vi "TcpServer.vi"(10 "Port in (0)":u16, 11 "IpAddress (127.0.0.1)":string="127.0.0.1") -> (0 "error out":errorcluster, 2 "Log":string, 3 "Port out":u16)   [LabVIEW 2022 SP3]
uses:
  TcpSocket/TcpServer/TcpServer.lvclass
  TcpSocket/Connection/Connection.lvclass
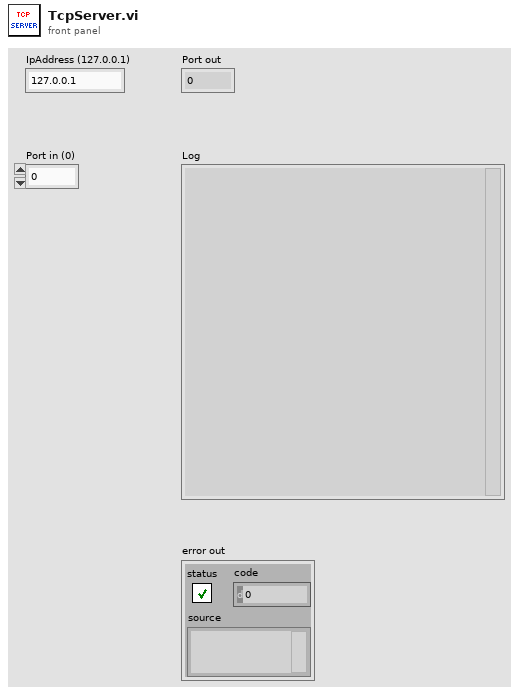
[diagram p1: front panel]
types:
  T1 = enum16{"Standard", "Buffered", "CRLF", "Immediate"}
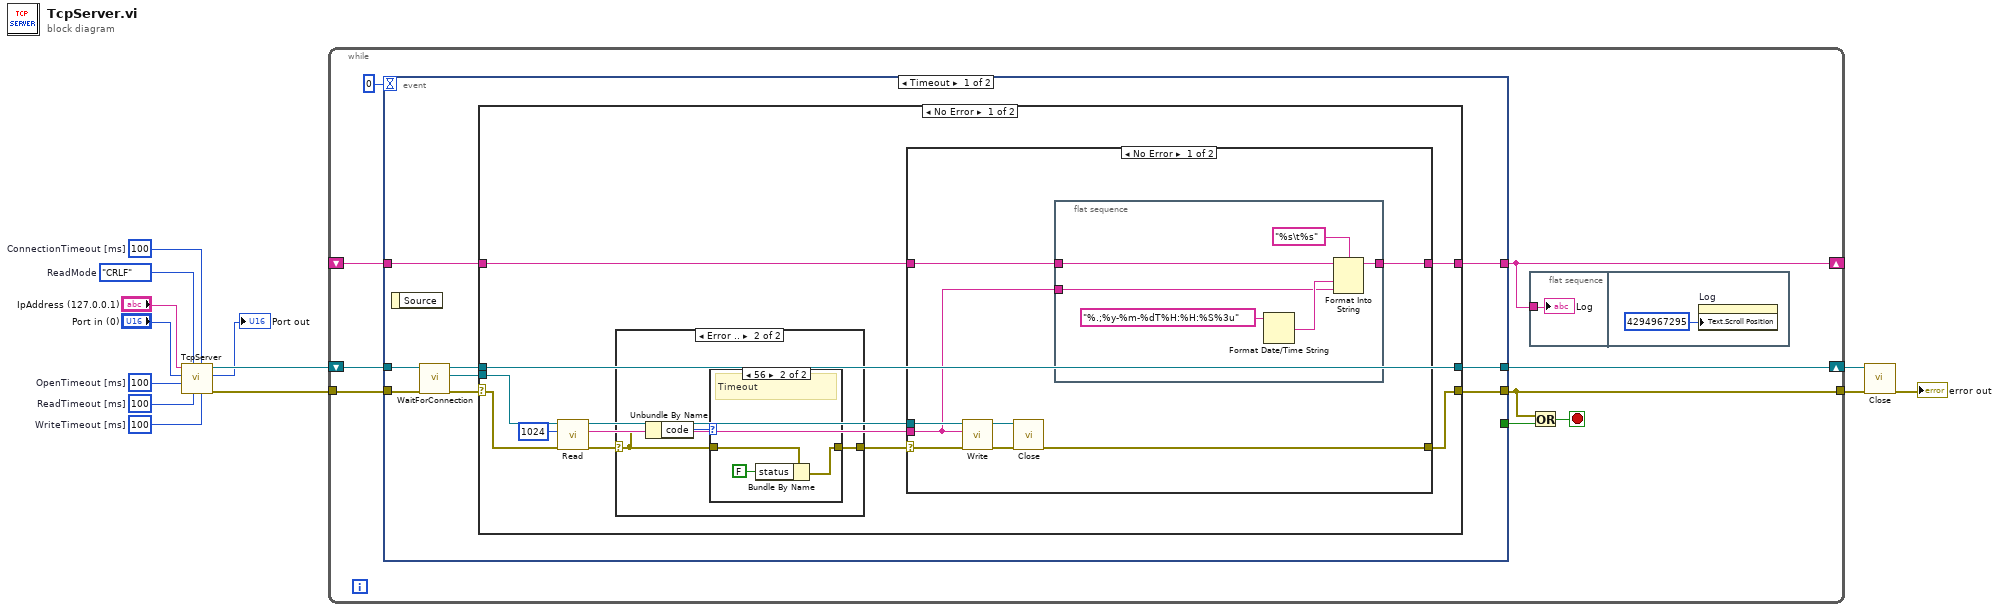
[diagram p0: block diagram]
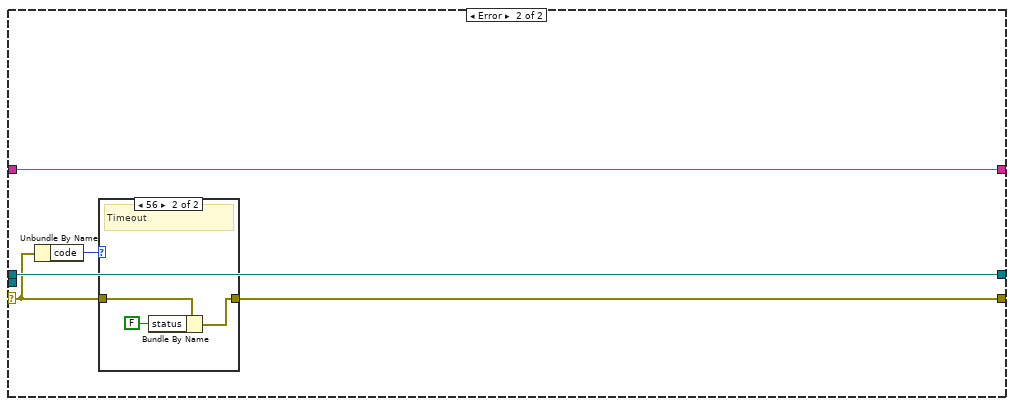
[diagram p5: hidden frame]
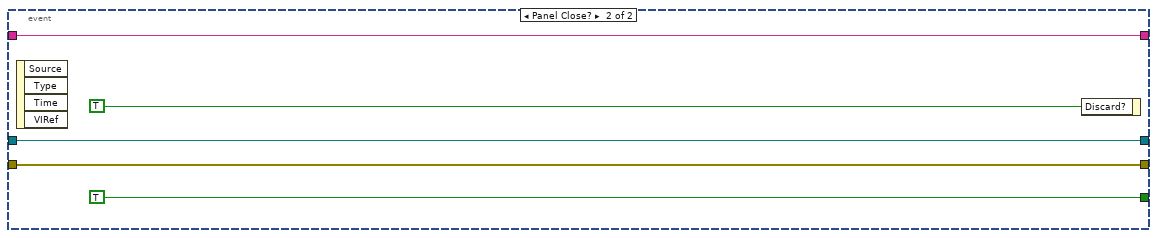
[diagram p7: hidden frame]
diagram:
  w1 = 100  # WriteTimeout [ms]
  w3 = 100  # ReadTimeout [ms]
  w6 = 100  # OpenTimeout [ms]
  w2 = 100  # ConnectionTimeout [ms]
  w7 = T1."CRLF"  # ReadMode
  n1 = call "TcpServer.vi"("WriteTimeout [ms] (5000)"=w1, "ConnectionTimeout [ms] (5000)"=w2, "ReadTimeout [ms] (5000)"=w3, "ReadMode (Standard)"=w7, "OpenTimeout [ms] (5000)"=w6, "Port in (0)"="Port in (0)", "IpAddress (127.0.0.1)"="IpAddress (127.0.0.1)") -> ("error out"=w11:errorcluster, "Port out"=→"Port out":u16, "TcpServer"=w5:refnum<class "TcpServer.lvclass">)  [unwired: 2 in]
  n2 = while {
    tunnel: w11 -> [w22]
    shift-right: [w20] -> w8
    shift-left: w5 -> [w21]
    tunnel: [w17] -> w10
    shift-right: [w14] -> _
    shift-left: _ -> [w15]
    stop <- w18 stop-if-true
    n3 = event shown="[0] Timeout" {
      selector: _ -> [_ _]
      dyn-events: _ -> [_ _]
      timeout: 0 -> [_ _]
      tunnel: w22 -> [w33 w81]
      tunnel: w21 -> [w32 w82]
      tunnel: [w30 w82] -> w20
      tunnel: [w28 w81] -> w17
      tunnel: [_ TRUE] -> w19
      tunnel: w15 -> [w27 w78]
      tunnel: [w26 w78] -> w14
      event Timeout {
        n4 = event-data() -> ()  [unwired: 1 in, 1 out]
        n5 = call-dynamic "WaitForConnection.vi"("error in (no error)"=w33, "TcpServer in"=w32) -> ("error out"=w25:errorcluster, "Connection"=w31:refnum<class "Connection.lvclass">, "TcpServer out"=w29:refnum<class "TcpServer.lvclass">)  [unwired: 7 in]
        n6 = case shown="No Error" w25 {
          selector: w25 -> [w40 w70]
          tunnel: w31 -> [w42 _]
          tunnel: [w44 w73] -> w30
          tunnel: w29 -> [w44 w73]
          tunnel: [w43 w69] -> w28
          tunnel: w27 -> [w36 w72]
          tunnel: [w37 w72] -> w26
          frame No Error {
            n7 = call-dynamic "Read.vi"("error in (no error)"=w40, "BytesToRead"=1024, "Connection in"=w42) -> ("error out"=w35:errorcluster, "Data"=w39:string, "Connection out"=w41:refnum<class "Connection.lvclass">)  [unwired: 6 in]
            n8 = case shown="Error .." w35 {
              selector: w35 -> [w61 w63]
              tunnel: [w61 w62] -> w34
              frame No Error {
              }
              frame Error {
                n9 = Unbundle By Name(w63) -> ("code"=w64:i32)
                n10 = case shown="56" w64 {
                  tunnel: w63 -> [w65 w68]
                  tunnel: [w65 w66] -> w62
                  frame Default {
                  }
                  frame 56 {
                    # "Timeout"
                    n11 = Bundle By Name(cluster=w68, "status"=FALSE) -> (w66:errorcluster)
                  }
                }
              }
            }
            n12 = case shown="No Error" w34 {
              selector: w34 -> [w45 w60]
              tunnel: [w52 w60] -> w43
              tunnel: w41 -> [w51 _]
              tunnel: w39 -> [w50 _]
              tunnel: [w49 w59] -> w37
              tunnel: w36 -> [w48 w59]
              frame No Error {
                n13 = call-dynamic "Write.vi"("error in (no error)"=w45, "Data"=w50, "Connection in"=w51) -> ("error out"=w46:errorcluster, "Connection out"=w47:refnum<class "Connection.lvclass">)  [unwired: 7 in]
                n14 = call-dynamic "Close.vi"("error in (no error)"=w46, "Connection"=w47) -> ("error out"=w52:errorcluster)  [unwired: 9 in]
                n15 = flat-sequence {
                  tunnel: w50 -> [w55]
                  tunnel: [w54] -> w49
                  tunnel: w48 -> [w53]
                  frame #0 {
                    n16 = Format Date/Time String(time format string (%c)="%.;%y-%m-%dT%H:%H:%S%3u") -> (date/time string=w58:string)  [unwired: 2 in]
                    n17 = Format Into String(format string="%s\t%s", initial string=w53, w58, w55) -> (resulting string=w54:string)  [unwired: 1 in, 1 out]
                  }
                }
              }
              frame Error {
              }
            }
          }
          frame Error {
            n18 = Unbundle By Name(w70) -> ("code"=w71:i32)
            n19 = case shown="56" w71 {
              tunnel: w70 -> [w74 w77]
              tunnel: [w74 w75] -> w69
              frame Default {
              }
              frame 56 {
                # "Timeout"
                n20 = Bundle By Name(cluster=w77, "status"=FALSE) -> (w75:errorcluster)
              }
            }
          }
        }
      }
      event Panel Close? {
        n21 = event-data() -> ()  [unwired: 1 in, 4 out]
        n22 = event-data("Discard?"=TRUE) -> ()  [unwired: 1 in, 1 out]
      }
    }
    n23 = flat-sequence {
      tunnel: w14 -> [w23]
      frame #0 {
        "Log" <- w23
      }
      frame #1 {
        n24 = property on="Log" class="Str"("Text.Scroll Position"=u32 4294967295) -> ()  [unwired: 2 in, 2 out]
      }
    }
    n25 = Or(x=w17, y=w19) -> (x .or. y?=w18:bool)
  }
  n26 = call-dynamic "Close.vi"("error in (no error)"=w10, "TcpSocket in"=w8) -> ("error out"=→"error out":errorcluster)  [unwired: 8 in, 1 out]
